vi "ShutterManual.vi"(8 "Error In":errorcluster, 11 "Manual Shutter in":T4) -> (0 "Error Out":errorcluster, 3 "Shutters out":T1)   [LabVIEW 2016]
uses:
  Controls/Shutter Manual.ctl
  Controls/Shutters.ctl
  Controls/Shutter Data.ctl
  Controls/Shutter States.ctl
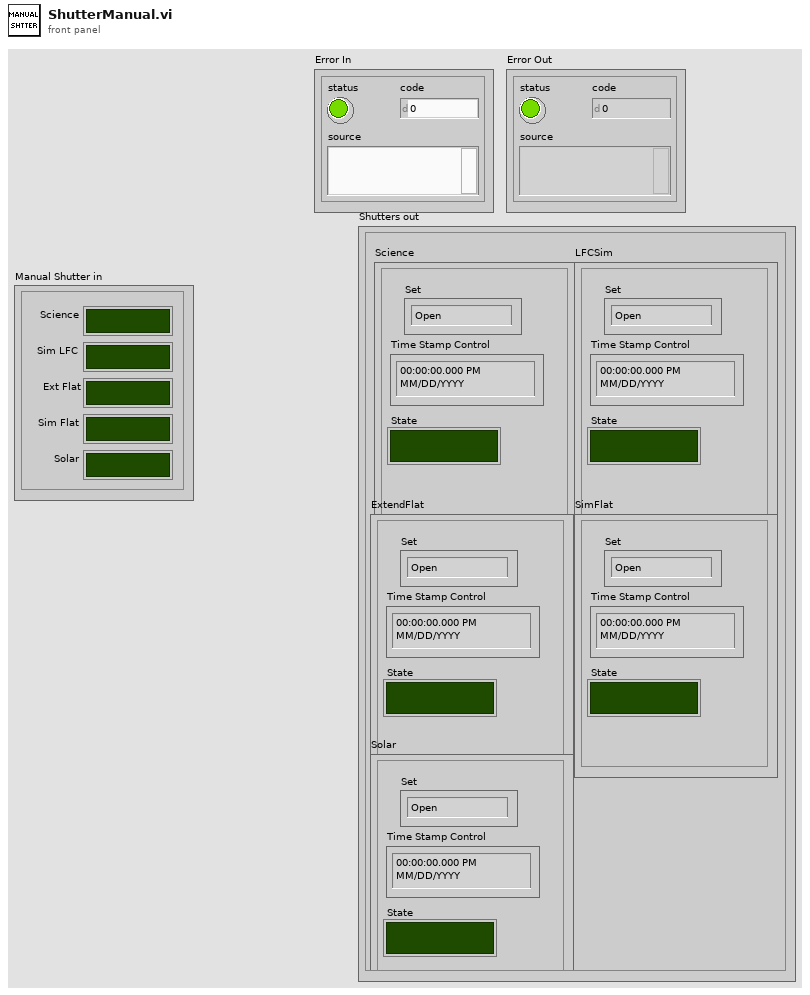
[diagram p1: front panel]
types:
  T1 = typedef "Shutters.ctl" = cluster{"Science":T2, "LFCSim":T2, "ExtendFlat":T2, "SimFlat":T2, "Solar":T2}
  T2 = typedef "Shutter Data.ctl" = cluster{"Time Stamp Control":timestamp, "State":bool, "Set":T3}
  T3 = typedef "Shutter States.ctl" = enum16{"Open", "Close", "Wait", "Off", "Arm", "Idle"}
  T4 = typedef "Shutter Manual.ctl" = cluster{"Science":bool, "Solar":bool, "Ext Flat":bool, "Sim LFC":bool, "Sim Flat":bool}
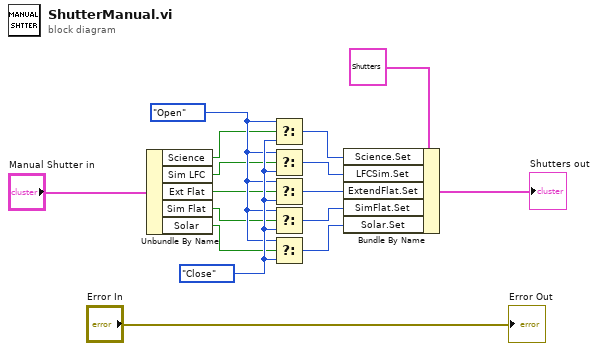
[diagram p0: block diagram]
diagram:
  w16 = Shutter_States."Close" ("Set")
  w15 = Shutter_States."Open" ("Set")
  n1 = Unbundle By Name("Manual Shutter in") -> ("Science"=w10:bool, "Sim LFC"=w11:bool, "Ext Flat"=w12:bool, "Sim Flat"=w13:bool, "Solar"=w14:bool)
  n2 = Select(t=w15, s=w10, f=w16) -> (s? t:f=w1:T3)
  n3 = Select(t=w15, s=w11, f=w16) -> (s? t:f=w5:T3)
  n4 = Select(t=w15, s=w12, f=w16) -> (s? t:f=w6:T3)
  n5 = Select(t=w15, s=w13, f=w16) -> (s? t:f=w7:T3)
  n6 = Select(t=w15, s=w14, f=w16) -> (s? t:f=w8:T3)
  n7 = Bundle By Name(cluster=T1 {"Science"={"Time Stamp Control"=timestamp(0 s since 1904-01-01), "State"=FALSE, "Set"=enum."Open"}, "LFCSim"={"Time Stamp Control"=timestamp(0 s since 1904-01-01), "State"=FALSE, "Set"=enum."Open"}, "ExtendFlat"={"Time Stamp Control"=timestamp(0 s since 1904-01-01), "State"=FALSE, "Set"=enum."Open"}, "SimFlat"={"Time Stamp Control"=timestamp(0 s since 1904-01-01), "State"=FALSE, "Set"=enum."Open"}, "Solar"={"Time Stamp Control"=timestamp(0 s since 1904-01-01), "State"=FALSE, "Set"=enum."Open"}} ("Shutters"), "Science.Set"=w1, "LFCSim.Set"=w5, "ExtendFlat.Set"=w6, "SimFlat.Set"=w7, "Solar.Set"=w8) -> (→"Shutters out":T1)
  "Error Out" <- "Error In"
